vi "LED_control.vi"() -> ()   [LabVIEW 2018]
uses:
  <instrlib>/niDMM/nidmm.llb/niDMM Function.ctl
  <instrlib>/niDMM/nidmm.llb/niDMM Resolution in Digits.ctl
  <instrlib>/niDCPower/nidcpower.llb/niDCPower Measurement Type.ctl
  <vilib>/Instr/_visa.llb/VISA Configure Serial Port (Instr).vi
  <instrlib>/niDMM/nidmm.llb/niDMM Configure Measurement Digits.vi
panel:
  in  "Записать":bool
  in  "Command":string="led_on"
  in  "Arduino":refnum<visa-resource-name>="COM3"
  out "NI DMM 1 Current 3":dbl caption="Current" format="%_6g"
  out "NI DMM 1 Current Char 3":dbl(graph)
  in  "NI DMM 1 units 3":string(combo)="1000000" caption="Units"
  out "Real Current, А":dbl format="%.5f"
  in  "NI DMM 1 Current Range 3":string(combo)="-1" caption="Range"
  out "currentmes_1, A":dbl caption="measurement" format="%_6g"
  out "chart_1":dbl(graph)=7.760296185722101e-05 caption="Waveform Chart 5"
  in  "voltlevel_1, V":dbl=3.0 caption="voltage level" format="%_6p"
  in  "curlim_1, A":dbl=0.1 caption="current limit" format="%_6p"
  out "chart_0":dbl(graph)=0.10912787137551659 caption="Waveform Chart 5"
  out "chart_2":dbl(graph)=0.14149308240176237
  in  "voltlevel_2, V":dbl caption="voltage level" format="%_6p"
  out "currentmes_2, A":dbl caption="measurement" format="%_6g"
  out "currentmes_0, A":dbl caption="measurement" format="%_6g"
  in  "curlim_2, A":dbl=0.1 caption="current limit" format="%_6p"
  in  "curlim_0, A":dbl=0.1 caption="current limit" format="%_6p"
  in  "voltlevel_0, V":dbl=6.0 caption="voltage level" format="%_6p"
  in  "NI DMM 1":refnum<k15>="PXI1Slot3"
  in  "Стоп":bool
  in  "Resource Name":refnum<k15>="PXI1Slot2" caption="Первый источник"
  in  "Питание":bool
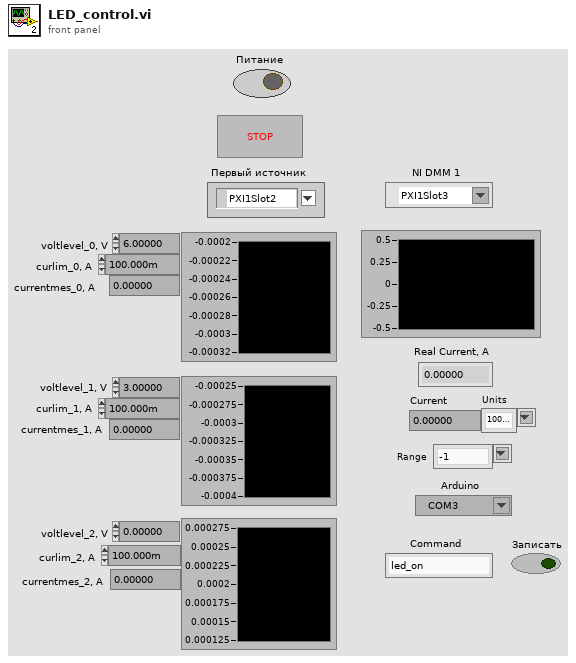
[diagram p1: front panel]
types:
  T1 = typedef "niDMM Function.ctl" = enum16{"DC Volts", "AC Volts", "DC Current", "AC Current", "2-wire Resistance", "4-wire Resistance", "Diode", "Frequency", "Period", "AC Volts DC Coupled", "Capacitance", "Inductance", "Temperature"}
  T2 = typedef "niDMM Resolution in Digits.ctl" = dbl
  T3 = typedef "niDCPower Measurement Type.ctl" = i32
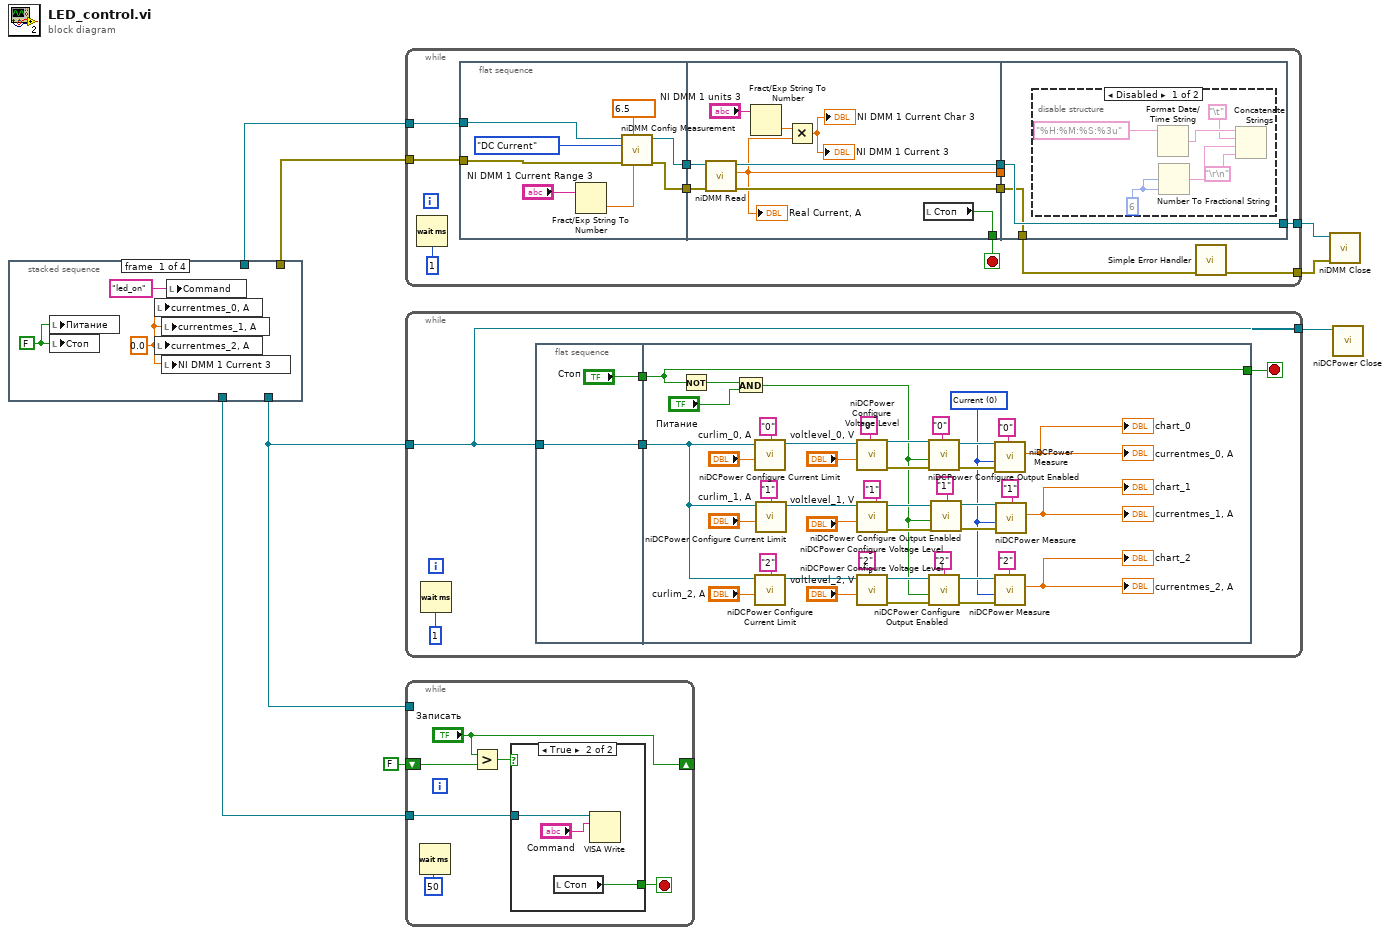
[diagram p0: block diagram]
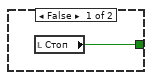
[diagram p2: hidden frame]
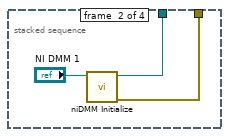
[diagram p4: hidden frame]
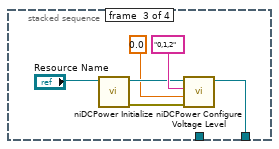
[diagram p5: hidden frame]
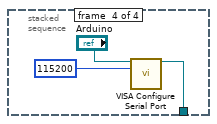
[diagram p6: hidden frame]
diagram:
  n1 = stacked-sequence {
    tunnel: [_ _ w17 _] -> w2
    tunnel: [_ w13 _ _] -> w7
    tunnel: [_ w12 _ _] -> w6
    tunnel: [_ _ _ w21] -> w1
    frame #0 {
      w10 = 0.0 ("currentmes_2")
      w11 = FALSE ("Стоп")
      n2 = local write "Питание"(w11) -> ()
      n3 = local write "Стоп"(w11) -> ()
      n4 = local write "currentmes_0, A"(w10) -> ()
      n5 = local write "currentmes_2, A"(w10) -> ()
      n6 = local write "currentmes_1, A"(w10) -> ()
      n7 = local write "NI DMM 1 Current 3"(w10) -> ()
      n8 = local write "Command"("led_on" ("Command 2")) -> ()
    }
    frame #1 {
      n9 = call <instrlib>:"niDMM Initialize.vi"("Instrument Descriptor"="NI DMM 1") -> ("error out"=w13:errorcluster, "instrument handle out"=w12:refnum<k15>)  [unwired: 9 in]
    }
    frame #2 {
      n10 = call <instrlib>:"niDCPower Initialize.vi"("resource name"="Resource Name") -> ("error out"=w16:errorcluster, "instrument handle out"=w18:refnum<k15>)  [unwired: 3 in, 6 out]
      n11 = call <instrlib>:"niDCPower Configure Voltage Level.vi"("error in (no error)"=w16, "voltage level"=0.0, "channel name"="0,1,2", "instrument handle"=w18) -> ("instrument handle out"=w17:refnum<k15>)  [unwired: 6 in, 1 out]
    }
    frame #3 {
      n12 = call-poly "VISA Configure Serial Port"("VISA resource name"="Arduino", "baud rate (9600)"=u32 115200) -> ("VISA resource name out"=w21:refnum<visa-resource-name>)  [unwired: 12 in, 1 out]
    }
  }
  n13 = while {
    tunnel: [w33] -> w5
    tunnel: [w29] -> w4
    tunnel: w6 -> [w26]
    tunnel: w7 -> [w25]
    stop <- w24 stop-if-true
    n14 = Wait (ms)(milliseconds to wait=u32 1) -> ()  [unwired: 1 out]
    n15 = flat-sequence {
      tunnel: [w40] -> w35
      tunnel: w26 -> [w38]
      tunnel: w25 -> [w42]
      tunnel: [w39] -> w32
      tunnel: w35 -> [w46]
      tunnel: [w51] -> w34
      tunnel: w32 -> [w50]
      tunnel: [w49] -> w31
      tunnel: [w45] -> w28
      tunnel: [w44] -> w24
      tunnel: w34 -> [w54]
      tunnel: [w54] -> w33
      tunnel: w31 -> [w53]
      tunnel: [w53] -> w30
      tunnel: w28 -> [_]
      frame #0 {
        w36 = T2 6.5 items=["3 1/2"=3.5, "4 1/2"=4.5, "5 1/2"=5.5, "6 1/2"=6.5, "7 1/2"=7.5] ("Resolution in Digits")
        n16 = Fract/Exp String To Number(string="NI DMM 1 Current Range 3") -> (number=w41:dbl)  [unwired: 3 in, 1 out]
        n17 = call-poly <instrlib>:"niDMM Config Measurement.vi"("Range"=w41, "Resolution in Digits"=w36, "error in (no error)"=w42, "Function"=niDMM_Function."DC Current" ("Measurement Type"), "instrument handle"=w38) -> ("error out"=w39:errorcluster, "instrument handle out"=w40:refnum<k15>)  [unwired: 5 in]
      }
      frame #1 {
        n18 = call <instrlib>:"niDMM Read.vi"("error in (no error)"=w50, "instrument handle"=w46) -> ("error out"=w49:errorcluster, "Measurement"=w45:dbl, "instrument handle out"=w51:refnum<k15>)  [unwired: 7 in]
        "Real Current, А" <- w45
        n19 = Fract/Exp String To Number(string="NI DMM 1 units 3") -> (number=w47:dbl)  [unwired: 3 in, 1 out]
        n20 = Multiply(x=w47, y=w45) -> (x*y=→"NI DMM 1 Current 3" →"NI DMM 1 Current Char 3":dbl)
        n21 = local read "Стоп"() -> (w44:bool)
      }
      frame #2 {
        n22 = disable-structure shown="Disabled" {
          frame Disabled {
            w60 = 6
            n23 = Format Date/Time String(time format string (%c)="%H:%M:%S:%3u") -> (date/time string=w58:string)  [unwired: 2 in]
            n24 = Number To Fractional String(width (-)=w60, precision (6)=w60) -> (F-format string=w56:string)  [unwired: 2 in]
            n25 = Concatenate Strings(w58, "\t", w56, "\r\n") -> ()  [unwired: 1 out]
          }
          frame Enabled {
          }
        }
      }
    }
    n26 = call <vilib>:"Simple Error Handler.vi"("error in (no error)"=w30) -> ("error out"=w29:errorcluster)  [unwired: 1 in, 7 out]
  }
  n27 = while {
    tunnel: w2 -> [w61]
    tunnel: [w61] -> w8
    stop <- w62 stop-if-true
    n28 = Wait (ms)(milliseconds to wait=u32 1) -> ()  [unwired: 1 out]
    n29 = flat-sequence {
      tunnel: w61 -> [w67]
      tunnel: [w67] -> w64
      tunnel: ["Стоп"] -> w63
      tunnel: w64 -> [w75]
      tunnel: w63 -> [w109]
      tunnel: [w109] -> w62
      frame #0 {
      }
      frame #1 {
        w74 = T3 0 items=["Current", "Voltage"] ("measurement type")
        n30 = Not(x=w109) -> (.not. x?=w108:bool)
        n31 = And(x=w108, y="Питание") -> (x .and. y?=w70:bool)
        n32 = call <instrlib>:"niDCPower Configure Current Limit.vi"("current limit"="curlim_0, A", "channel name"="0", "instrument handle"=w75) -> ("instrument handle out"=w94:refnum<k15>)  [unwired: 7 in, 1 out]
        n33 = call <instrlib>:"niDCPower Configure Current Limit.vi"("current limit"="curlim_2, A", "channel name"="2", "instrument handle"=w75) -> ("instrument handle out"=w93:refnum<k15>)  [unwired: 7 in, 1 out]
        n34 = call <instrlib>:"niDCPower Configure Current Limit.vi"("current limit"="curlim_1, A", "channel name"="1", "instrument handle"=w75) -> ("instrument handle out"=w102:refnum<k15>)  [unwired: 7 in, 1 out]
        n35 = call <instrlib>:"niDCPower Configure Voltage Level.vi"("voltage level"="voltlevel_0, V", "channel name"="0", "instrument handle"=w94) -> ("error out"=w99:errorcluster, "instrument handle out"=w96:refnum<k15>)  [unwired: 7 in]
        n36 = call <instrlib>:"niDCPower Configure Voltage Level.vi"("voltage level"="voltlevel_1, V", "channel name"="1", "instrument handle"=w102) -> ("error out"=w105:errorcluster, "instrument handle out"=w103:refnum<k15>)  [unwired: 7 in]
        n37 = call <instrlib>:"niDCPower Configure Voltage Level.vi"("voltage level"="voltlevel_2, V", "channel name"="2", "instrument handle"=w93) -> ("error out"=w98:errorcluster, "instrument handle out"=w97:refnum<k15>)  [unwired: 7 in]
        n38 = call <instrlib>:"niDCPower Configure Output Enabled.vi"("error in (no error)"=w99, "output enabled"=w70, "channel name"="0", "instrument handle"=w96) -> ("error out"=w89:errorcluster, "instrument handle out"=w90:refnum<k15>)  [unwired: 6 in]
        n39 = call <instrlib>:"niDCPower Configure Output Enabled.vi"("error in (no error)"=w98, "output enabled"=w70, "channel name"="2", "instrument handle"=w97) -> ("error out"=w88:errorcluster, "instrument handle out"=w87:refnum<k15>)  [unwired: 6 in]
        n40 = call <instrlib>:"niDCPower Configure Output Enabled.vi"("error in (no error)"=w105, "output enabled"=w70, "channel name"="1", "instrument handle"=w103) -> ("error out"=w106:errorcluster, "instrument handle out"=w104:refnum<k15>)  [unwired: 6 in]
        n41 = call <instrlib>:"niDCPower Measure.vi"("error in (no error)"=w89, "measurement type"=w74, "channel name"="0", "instrument handle"=w90) -> ("measurement"=→"currentmes_0, A" →"chart_0":dbl)  [unwired: 5 in, 2 out]
        n42 = call <instrlib>:"niDCPower Measure.vi"("error in (no error)"=w88, "measurement type"=w74, "channel name"="2", "instrument handle"=w87) -> ("measurement"=→"currentmes_2, A" →"chart_2":dbl)  [unwired: 5 in, 2 out]
        n43 = call <instrlib>:"niDCPower Measure.vi"("error in (no error)"=w106, "measurement type"=w74, "channel name"="1", "instrument handle"=w104) -> ("measurement"=→"chart_1" →"currentmes_1, A":dbl)  [unwired: 5 in, 2 out]
      }
    }
  }
  n44 = while {
    tunnel: w1 -> [w115]
    shift-right: ["Записать"] -> _
    shift-left: FALSE ("Записать") -> [w112]
    tunnel: w2 -> [_]
    stop <- w113 stop-if-true
    n45 = Wait (ms)(milliseconds to wait=u32 50) -> ()  [unwired: 1 out]
    n46 = Greater?(x="Записать", y=w112) -> (0:w110:bool)
    n47 = case shown="True" w110 {
      tunnel: w115 -> [_ w119]
      tunnel: [w116 w118] -> w113
      frame False {
        n48 = local read "Стоп"() -> (w116:bool)
      }
      frame True {
        n49 = local read "Стоп"() -> (w118:bool)
        n50 = VISA Write(VISA resource name=w119, write buffer="Command") -> ()  [unwired: 1 in, 3 out]
      }
    }
  }
  n51 = call <instrlib>:"niDMM Close.vi"("error in (no error)"=w4, "instrument handle"=w5) -> ()  [unwired: 9 in, 1 out]
  n52 = call <instrlib>:"niDCPower Close.vi"("instrument handle"=w8) -> ()  [unwired: 10 in, 1 out]
